vi "Write Table of Content.vi"(0 "PDF Report IN":refnum<class "PDF Report Class.lvclass">=refnum, 11 "error in (no error)":errorcluster) -> (4 "PDF Report OUT":refnum<class "PDF Report Class.lvclass">, 8 "TOC page":cluster{"Start":i32, "Number":i32}, 15 "error out":errorcluster)   [LabVIEW 2019]
doc: "Version 1.12.0\nDeveloped by Jean-Marc Simard\nCopyright © 2013, Exaprom Inc.\nAll rights reserved.\nLicense: BSD\n\nWith iTextSharp 4.1.6 (http://itextsharp.sourceforge.net)\nunder Mozilla Public License Version 1.1\n(http://www.mozilla.org/MPL/MPL-1.1.html)"
uses:
  <userlib>/Exaprom PDF/LV Class/PDF Report Class/PDF Report Class.lvclass
  <userlib>/Exaprom PDF/LV Class/Fonts Class/Font Class.lvclass
  <userlib>/Exaprom PDF/LV Class/Header and Footer Class/Header and Footer Class.lvclass
  <userlib>/Exaprom PDF/Controls/Initialization Controls/Defaut Paragraphe and Line Spacing.ctl
  <userlib>/Exaprom PDF/Controls/Text Controls/Texte alignement.ctl
  <userlib>/Exaprom PDF/Controls/Text Controls/Line spacing.ctl
  C:/Program Files/National Instruments/LabVIEW 2019/user.lib/Exaprom PDF/DLL/itextsharp.dll
  DLL/itextsharp.dll
  <userlib>/Exaprom PDF/Controls/Font Controls/Font size.ctl
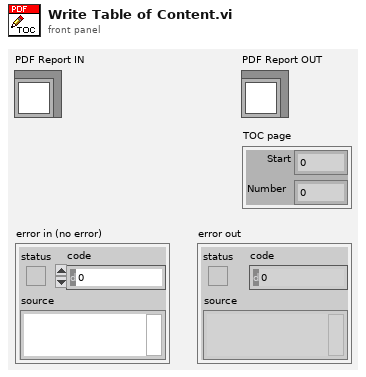
[diagram p1: front panel]
types:
  T1 = typedef "Defaut Paragraphe and Line Spacing.ctl" = cluster{" Aligment":T2, "Line spacing":T3}
  T2 = typedef "Texte alignement.ctl" = enum16{"Select", "CENTER", "JUSTIFY", "LEFT", "RIGHT"}
  T3 = typedef "Line spacing.ctl" = enum16{"Select", "1.0", "1.5", "2.0"}
  T4 = typedef "Font size.ctl" = sgl
  T5 = typedef "TOC.ctl" = cluster{"Title":string, "Title Font":T6, "Chapter and section Font":T6, "First TOC page":u16, "Add TOC?":bool}
  T6 = typedef "Font complete cluster.ctl" = cluster{"Name":string, "Size":T4, "Color":T7, "Style":cluster{"Bold":bool, "Italic":bool, "Underline":bool, "Strikeout":bool}, "Type":T8}
  T7 = typedef "Font color.ctl" = u32
  T8 = typedef "Type and encoding.ctl" = cluster{"Type&direction":T9, "Embedded":bool, "Encoding":string}
  T9 = typedef "Type and run direction.ctl" = enum16{"Select", "ASCII", "UTF-16", "UTF-16 (default)", "UTF-16 (LTR)", "UTF-16 (RTL)"}
  T10 = typedef "TOC Line.ctl" = cluster{"Title":string, "Level":u16, "GoTo Page":u16, "GoTo Position":u16, "Destination":string, "Type & run direction":T9}
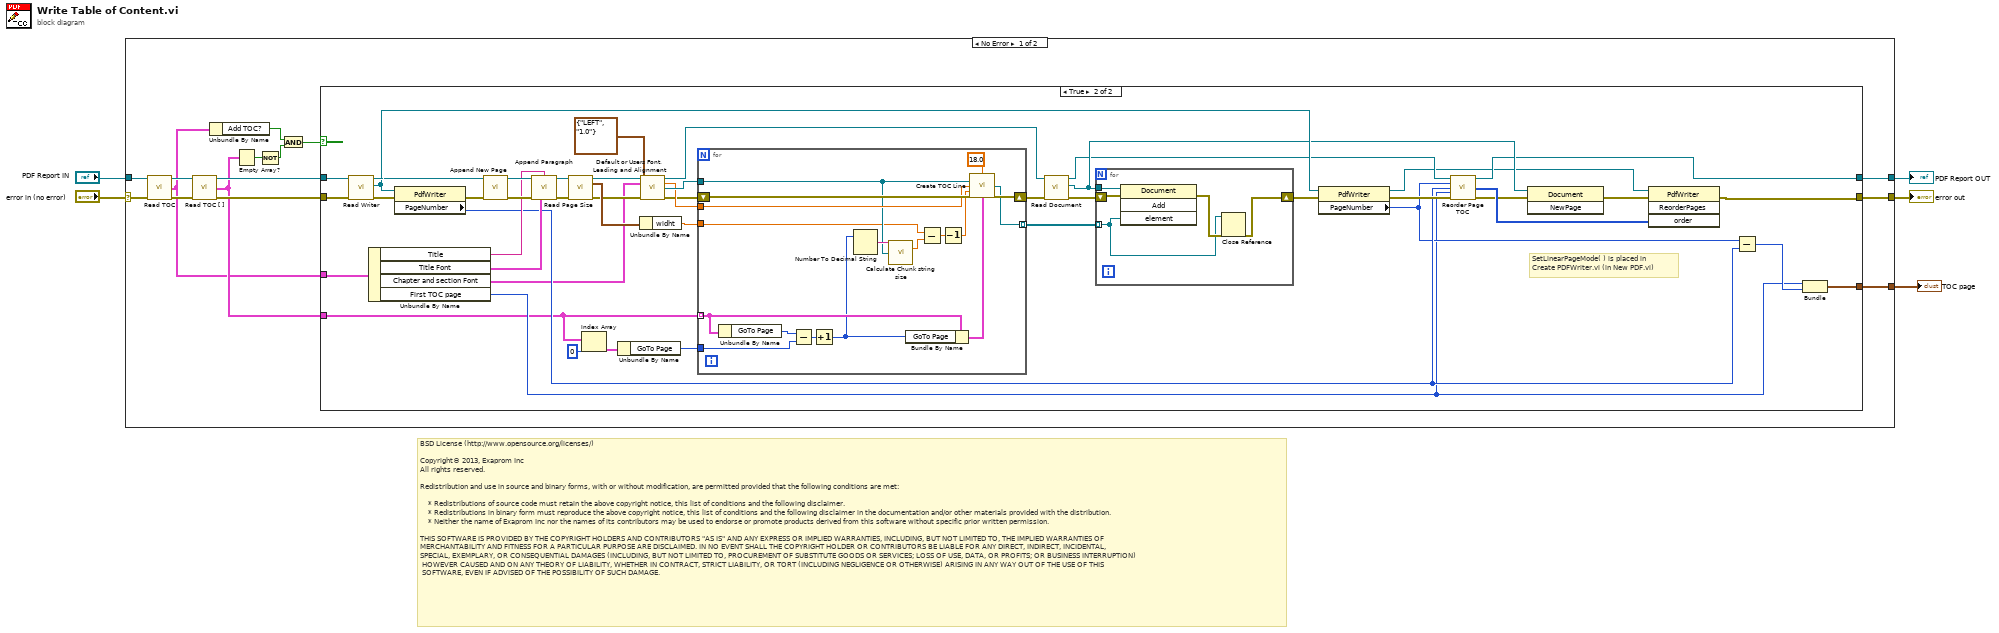
[diagram p0: block diagram]
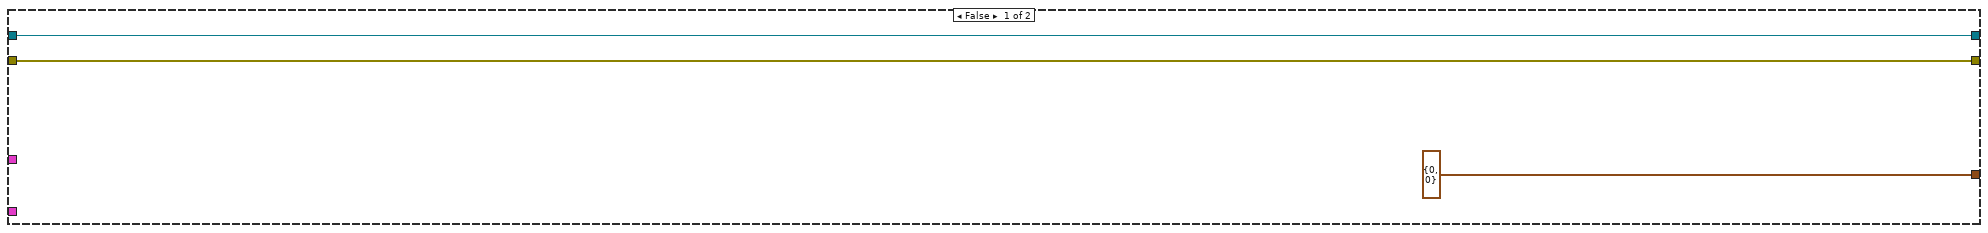
[diagram p2: hidden frame]
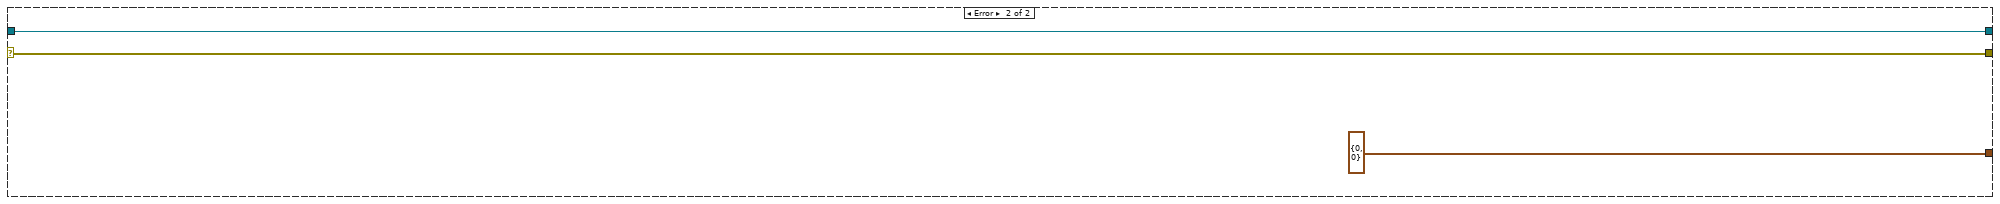
[diagram p3: hidden frame]
diagram:
  # "BSD License (http://www.opensource.org/licenses/)\n\nCopyright© 2013, Exaprom Inc\nAll rights reserved.\n\nRedistribution and use in source and binary forms, with or without modification, are permitted provided that the following conditions are met:\n\n    * Redistributions of source code must retain the above copyright notice, this list of conditions and the following disclaimer.\n    * Redistributions in binary form must reproduce the above copyright notice, this list of conditions and the following disclaimer in the documentation and/or other materials provided with the distribution.\n    * Neither the name of Exaprom Inc nor the names of its contributors may be used to endorse or promote products derived from this software without specific prior written permission.\n\nTHIS SOFTWARE IS PROVIDED BY THE COPYRIGHT HOLDERS AND CONTRIBUTORS \"AS IS\" AND ANY EXPRESS OR IMPLIED WARRANTIES, INCLUDING, BUT NOT LIMITED TO, THE IMPLIED WARRANTIES OF \nMERCHANTABILITY AND FITNESS FOR A PARTICULAR PURPOSE ARE DISCLAIMED. IN NO EVENT SHALL THE COPYRIGHT HOLDER OR CONTRIBUTORS BE LIABLE FOR ANY DIRECT, INDIRECT, INCIDENTAL,\nSPECIAL, EXEMPLARY, OR CONSEQUENTIAL DAMAGES (INCLUDING, BUT NOT LIMITED TO, PROCUREMENT OF SUBSTITUTE GOODS OR SERVICES; LOSS OF USE, DATA, OR PROFITS; OR BUSINESS INTERRUPTION)\n HOWEVER CAUSED AND ON ANY THEORY OF LIABILITY, WHETHER IN CONTRACT, STRICT LIABILITY, OR TORT (INCLUDING NEGLIGENCE OR OTHERWISE) ARISING IN ANY WAY OUT OF THE USE OF THIS\n SOFTWARE, EVEN IF ADVISED OF THE POSSIBILITY OF SUCH DAMAGE."
  n1 = case shown="No Error" "error in (no error)" {
    selector: "error in (no error)" -> [w7 w92]
    tunnel: "PDF Report IN" -> [w8 w93]
    tunnel: [w20 w93] -> w4
    tunnel: [w19 w92] -> w3
    tunnel: [w6 cluster{"PageNumber":i32, i32} {"PageNumber"=0, 0}] -> w1
    frame No Error {
      n2 = call-dynamic "Read TOC.vi"("PDF Report Class in"=w8, "error in (no error)"=w7) -> ("PDF Report Class out"=w15:refnum<class "PDF Report Class.lvclass">, "TOC"=w9:T5, "error out"=w14:errorcluster)  [unwired: 11 in]
      n3 = call-dynamic "Read TOC [ ].vi"("PDF Report Class in"=w15, "error in (no error)"=w14) -> ("PDF Report Class out"=w18:refnum<class "PDF Report Class.lvclass">, "TOC [ ]"=w16:T10[], "error out"=w17:errorcluster)  [unwired: 11 in]
      n4 = Unbundle By Name(w9) -> ("Add TOC?"=w11:bool)
      n5 = Empty Array?(array=w16) -> (empty?=w13:bool)
      n6 = Not(x=w13) -> (.not. x?=w12:bool)
      n7 = And(x=w11, y=w12) -> (x .and. y?=w10:bool)
      n8 = case shown="True" w10 {
        tunnel: [w23 w39] -> w20
        tunnel: [w22 w35] -> w19
        tunnel: w18 -> [w23 w59]
        tunnel: w17 -> [w22 w56]
        tunnel: w16 -> [_ w27]
        tunnel: w9 -> [_ w50]
        tunnel: [cluster{"PageNumber":i32, i32} {"PageNumber"=0, 0} w32] -> w6
        frame False {
        }
        frame True {
          # "SetLinearPageMode( ) is placed in\nCreate PDFWriter.vi (in New PDF.vi)"
          n9 = call-dynamic "Read Writer.vi"("error in (no error)"=w56, "PDF Report Class in"=w59) -> ("error out"=w55:errorcluster, "Writer"=w44:refnum<k24>, "PDF Report Class out"=w57:refnum<class "PDF Report Class.lvclass">)  [unwired: 7 in]
          n10 = Unbundle By Name(w50) -> ("Title"=w49:string, "Title Font"=w47:T6, "Chapter and section Font"=w28:T6, "First TOC page"=w29:u16)
          n11 = property class="PdfWriter"(reference=w44, error in=w55) -> (error out=w54:errorcluster, "PageNumber"=w36:i32)  [unwired: 1 out]
          n12 = call <userlib>:"Append New Page.vi"("PDF Report"=w57, "error in (no error)"=w54) -> ("PDF Report duplicate"=w58:refnum<class "PDF Report Class.lvclass">, "error OUT"=w52:errorcluster)  [unwired: 12 in]
          n13 = call <userlib>:"Append Paragraph.vi"("PDF Report"=w58, "Text"=w49, "error in (no error)"=w52, "Font"=w47) -> ("PDF Report duplicate"=w53:refnum<class "PDF Report Class.lvclass">, "error out"=w51:errorcluster)  [unwired: 10 in]
          n14 = call <userlib>:"Read Page Size.vi"("PDF Report"=w53, "error in (no error)"=w51) -> ("PDF Report duplicate"=w30:refnum<class "PDF Report Class.lvclass">, "Text zone (points)"=w62:cluster{"widht":sgl, "height":sgl}, "error out"=w31:errorcluster)  [unwired: 10 in, 1 out]
          n15 = Index Array(array=w27, index=0) -> (element=w26:T10)
          n16 = Unbundle By Name(w26) -> ("GoTo Page"=w24:u16)
          n17 = Unbundle By Name(w62) -> ("widht"=w61:sgl)
          n18 = call <userlib>:"Default or Users Font, Leading and Alignment.vi"("PDF Report"=w30, "Font"=w28, "Paragraphe cluster"=T1 {" Aligment"=enum."LEFT", "Line spacing"=enum."1.0"}, "error in (no error)"=w31) -> ("PDF Report duplicate"=w60:refnum<class "PDF Report Class.lvclass">, "Leading"=w67:T4, "Font Ref"=w68:refnum<k24>, "error out"=w66:errorcluster)  [unwired: 5 in, 3 out]
          n19 = for {
            tunnel: w27 -> [w76] mode=indexing
            tunnel: w68 -> [w85]
            tunnel: w67 -> [w88]
            tunnel: w61 -> [w83]
            tunnel: [w87] -> w64 mode=indexing
            shift-right: [w89] -> w65
            shift-left: w66 -> [w90]
            tunnel: w24 -> [w78]
            n20 = Unbundle By Name(w76) -> ("GoTo Page"=w79:u16)
            n21 = Subtract(x=w79, y=w78) -> (x-y=w77:u16)
            n22 = Increment(x=w77) -> (x+1=w75:u16)
            n23 = Number To Decimal String(number=w75) -> (decimal integer string=w86:string)  [unwired: 1 in]
            n24 = call <userlib>:"Calculate Chunk string size.vi"("String"=w86, "Font refnum"=w85) -> ("Width"=w84:sgl)  [unwired: 10 in, 3 out]
            n25 = Bundle By Name(cluster=w76, "GoTo Page"=w75) -> (w74:T10)
            n26 = Subtract(x=w83, y=w84) -> (x-y=w82:sgl)
            n27 = Decrement(x=w82) -> (x-1=w81:sgl)
            n28 = call <userlib>:"Create TOC Line.vi"("Indentation (points)"=T4 18.0, "Font Ref"=w85, "Font Size"=w88, "Width (points)"=w81, "error in (no error)"=w90, "TOC Line"=w74) -> ("Paragraph"=w87:refnum<k24>, "error out"=w89:errorcluster)  [unwired: 7 in, 1 out]
          }
          n29 = call-dynamic "Read Document.vi"("error in (no error)"=w65, "PDF Report Class in"=w60) -> ("error out"=w63:errorcluster, "Document"=w43:refnum<k24>, "PDF Report Class out"=w41:refnum<class "PDF Report Class.lvclass">)  [unwired: 7 in]
          n30 = for {
            tunnel: w64 -> [w70] mode=indexing
            shift-right: [w69] -> w46
            shift-left: w63 -> [w73]
            tunnel: w43 -> [w72]
            n31 = invoke class="Document" method="Add"(reference=w72, error in=w73, "element"=w70) -> (error out=w71:errorcluster)  [unwired: 1 in, 3 out]
            n32 = Close Reference(reference=w70, error in (no error)=w71) -> (error out=w69:errorcluster)
          }
          n33 = property class="PdfWriter"(reference=w44, error in=w46) -> (reference out=w37:refnum<k24>, error out=w42:errorcluster, "PageNumber"=w34:i32)
          n34 = call <userlib>:"Reorder Page TOC.vi"("PDF Report IN"=w41, "Number pages after TOC"=w34, "Number pages before TOC"=w36, "TOC start at page"=w29, "error in (no error)"=w42) -> ("PDF Report OUT"=w39:refnum<class "PDF Report Class.lvclass">, "Pages [ ]"=w40:i32[], "error out"=w38:errorcluster)  [unwired: 8 in]
          n35 = invoke class="Document" method="NewPage"(reference=w43, error in=w38) -> (error out=w45:errorcluster)  [unwired: 1 in, 2 out]
          n36 = invoke class="PdfWriter" method="ReorderPages"(reference=w37, error in=w45, "order"=w40) -> (error out=w35:errorcluster)  [unwired: 1 in, 3 out]
          n37 = Subtract(x=w34, y=w36) -> (x-y=w33:i32)
          n38 = Bundle("First TOC page"=w29, w33) -> (w32:cluster{"First TOC page":u16, i32})  [unwired: 1 in]
        }
      }
    }
    frame Error {
    }
  }
  "PDF Report OUT" <- w4
  "error out" <- w3
  "TOC page" <- w1
